vi "DeviceNameChange.vi"(0 "软元件":string="D0") -> (1 "字符串":string, 2 "类型":string)   [LabVIEW 2018]
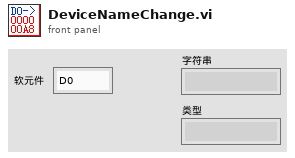
[diagram p1: front panel]
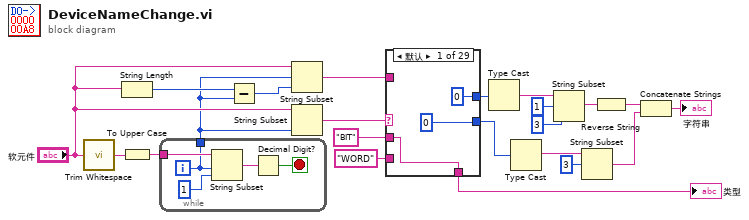
[diagram p0: block diagram]
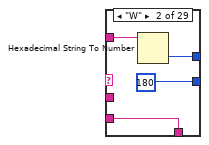
[diagram p2: hidden frame]
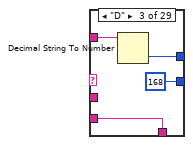
[diagram p3: hidden frame]
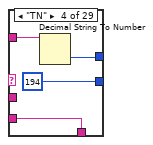
[diagram p4: hidden frame]
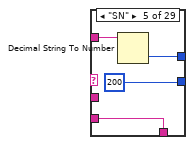
[diagram p5: hidden frame]
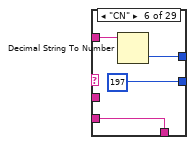
[diagram p6: hidden frame]
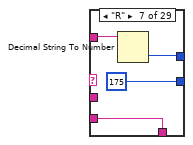
[diagram p7: hidden frame]
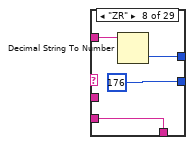
[diagram p8: hidden frame]
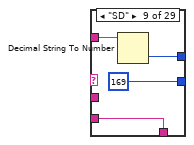
[diagram p9: hidden frame]
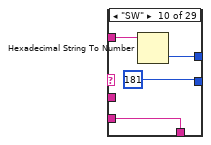
[diagram p10: hidden frame]
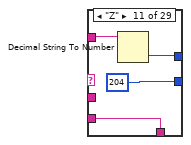
[diagram p11: hidden frame]
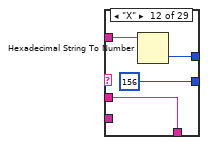
[diagram p12: hidden frame]
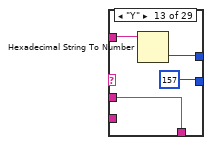
[diagram p13: hidden frame]
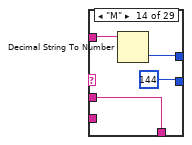
[diagram p14: hidden frame]
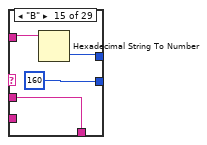
[diagram p15: hidden frame]
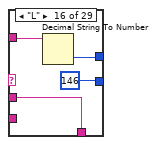
[diagram p16: hidden frame]
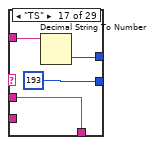
[diagram p17: hidden frame]
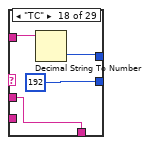
[diagram p18: hidden frame]
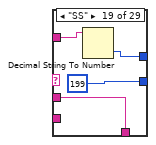
[diagram p19: hidden frame]
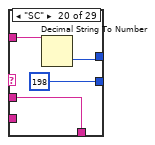
[diagram p20: hidden frame]
diagram:
  n1 = call <vilib>:"Trim Whitespace.vi"("string"="软元件") -> ("trimmed string"=w22:string)  [unwired: 1 in]
  n2 = String Length(string="软元件") -> (length=w18:i32)
  n3 = To Upper Case(1:w22) -> (0:w21:string)
  n4 = while {
    tunnel: w21 -> [w26]
    tunnel: [w23] -> w16
    i -> [w23]
    stop <- w24 stop-if-true
    n5 = String Subset(string=w26, offset (0)=w23, length (rest)=1 ("长度（剩余）")) -> (substring=w25:string)
    n6 = Decimal Digit?(1:w25) -> (0:w24:bool)
  }
  n7 = Subtract(x=w18, y=w16) -> (x-y=w17:i32)
  n8 = String Subset(string="软元件", offset (0)=w16, length (rest)=w17) -> (substring=w15:string)
  n9 = String Subset(string="软元件", length (rest)=w16) -> (substring=w20:string)  [unwired: 1 in]
  n10 = case shown="默认" w20 {
    tunnel: [0 180 168 194 200 197 175 176 169 181 204 156 157 144 160 146 193 192 199 198 196 195 161 145 152 162 163 147 148] -> w9
    tunnel: w15 -> [_ w33 w37 w41 w44 w49 w53 w57 w61 w65 w69 w73 w77 w81 w85 w89 w93 w97 w101 w105 w109 w113 w117 w121 w125 w129 w133 w137 w141]
    tunnel: [u32 0 w32 w36 w40 w45 w48 w52 w56 w60 w64 w68 w72 w76 w80 w84 w88 w92 w96 w100 w104 w108 w112 w116 w120 w124 w128 w132 w136 w140] -> w14
    tunnel: "BIT" -> [w28 _ _ _ _ _ _ _ _ _ _ w71 w75 w79 w83 w87 w91 w95 w99 w103 w107 w111 w115 w119 w123 w127 w131 w135 w139]
    tunnel: "WORD" -> [_ w31 w35 w39 w43 w47 w51 w55 w59 w63 w67 _ _ _ _ _ _ _ _ _ _ _ _ _ _ _ _ _ _]
    tunnel: [w28 w31 w35 w39 w43 w47 w51 w55 w59 w63 w67 w71 w75 w79 w83 w87 w91 w95 w99 w103 w107 w111 w115 w119 w123 w127 w131 w135 w139] -> w1
    frame Default {
    }
    frame "W" {
      n11 = Hexadecimal String To Number(string=w33) -> (number=w32:u32)  [unwired: 2 in, 1 out]
    }
    frame "D" {
      n12 = Decimal String To Number(string=w37) -> (number=w36:i32)  [unwired: 2 in, 1 out]
    }
    frame "TN" {
      n13 = Decimal String To Number(string=w41) -> (number=w40:i32)  [unwired: 2 in, 1 out]
    }
    frame "SN" {
      n14 = Decimal String To Number(string=w44) -> (number=w45:i32)  [unwired: 2 in, 1 out]
    }
    frame "CN" {
      n15 = Decimal String To Number(string=w49) -> (number=w48:i32)  [unwired: 2 in, 1 out]
    }
    frame "R" {
      n16 = Decimal String To Number(string=w53) -> (number=w52:i32)  [unwired: 2 in, 1 out]
    }
    frame "ZR" {
      n17 = Decimal String To Number(string=w57) -> (number=w56:i32)  [unwired: 2 in, 1 out]
    }
    frame "SD" {
      n18 = Decimal String To Number(string=w61) -> (number=w60:i32)  [unwired: 2 in, 1 out]
    }
    frame "SW" {
      n19 = Hexadecimal String To Number(string=w65) -> (number=w64:u32)  [unwired: 2 in, 1 out]
    }
    frame "Z" {
      n20 = Decimal String To Number(string=w69) -> (number=w68:i32)  [unwired: 2 in, 1 out]
    }
    frame "X" {
      n21 = Hexadecimal String To Number(string=w73) -> (number=w72:u32)  [unwired: 2 in, 1 out]
    }
    frame "Y" {
      n22 = Hexadecimal String To Number(string=w77) -> (number=w76:u32)  [unwired: 2 in, 1 out]
    }
    frame "M" {
      n23 = Decimal String To Number(string=w81) -> (number=w80:i32)  [unwired: 2 in, 1 out]
    }
    frame "B" {
      n24 = Hexadecimal String To Number(string=w85) -> (number=w84:u32)  [unwired: 2 in, 1 out]
    }
    frame "L" {
      n25 = Decimal String To Number(string=w89) -> (number=w88:i32)  [unwired: 2 in, 1 out]
    }
    frame "TS" {
      n26 = Decimal String To Number(string=w93) -> (number=w92:i32)  [unwired: 2 in, 1 out]
    }
    frame "TC" {
      n27 = Decimal String To Number(string=w97) -> (number=w96:i32)  [unwired: 2 in, 1 out]
    }
    frame "SS" {
      n28 = Decimal String To Number(string=w101) -> (number=w100:i32)  [unwired: 2 in, 1 out]
    }
    frame "SC" {
      n29 = Decimal String To Number(string=w105) -> (number=w104:i32)  [unwired: 2 in, 1 out]
    }
    frame "CS" {
      n30 = Decimal String To Number(string=w109) -> (number=w108:i32)  [unwired: 2 in, 1 out]
    }
    frame "CC" {
      n31 = Decimal String To Number(string=w113) -> (number=w112:i32)  [unwired: 2 in, 1 out]
    }
    frame "SB" {
      n32 = Hexadecimal String To Number(string=w117) -> (number=w116:u32)  [unwired: 2 in, 1 out]
    }
    frame "SM" {
      n33 = Decimal String To Number(string=w121) -> (number=w120:i32)  [unwired: 2 in, 1 out]
    }
    frame "S" {
      n34 = Decimal String To Number(string=w125) -> (number=w124:i32)  [unwired: 2 in, 1 out]
    }
    frame "DX" {
      n35 = Hexadecimal String To Number(string=w129) -> (number=w128:u32)  [unwired: 2 in, 1 out]
    }
    frame "DY" {
      n36 = Hexadecimal String To Number(string=w133) -> (number=w132:u32)  [unwired: 2 in, 1 out]
    }
    frame "F" {
      n37 = Decimal String To Number(string=w137) -> (number=w136:i32)  [unwired: 2 in, 1 out]
    }
    frame "V" {
      n38 = Decimal String To Number(string=w141) -> (number=w140:i32)  [unwired: 2 in, 1 out]
    }
  }
  "类型" <- w1
  n39 = Type Cast(x=w14) -> (*(type *) &x=w13:string)  [unwired: 1 in]
  n40 = Type Cast(x=w9) -> (*(type *) &x=w8:string)  [unwired: 1 in]
  n41 = String Subset(string=w13, offset (0)=1 ("偏移量(0)"), length (rest)=3 ("长度（剩余）")) -> (substring=w10:string)
  n42 = String Subset(string=w8, offset (0)=3 ("偏移量(0)")) -> (substring=w5:string)  [unwired: 1 in]
  n43 = Reverse String(1:w10) -> (0:w6:string)
  n44 = Concatenate Strings(w6, w5) -> (→"字符串":string)
